vi "TemperatureConverter.vi"() -> ()   [LabVIEW 2021]
panel:
  in  "(STOP)":bool
  out "Output":dbl
  in  "Input":dbl
  in  "MODE":T1(ring)
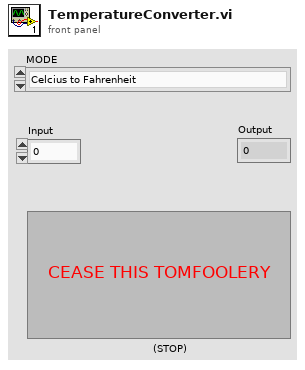
[diagram p1: front panel]
types:
  T1 = enum16{"Celcius to Fahrenheit", "Fahrenheit to Celcius", "Celcius to Kelvin", "Fahrenheit to Kelvin"}
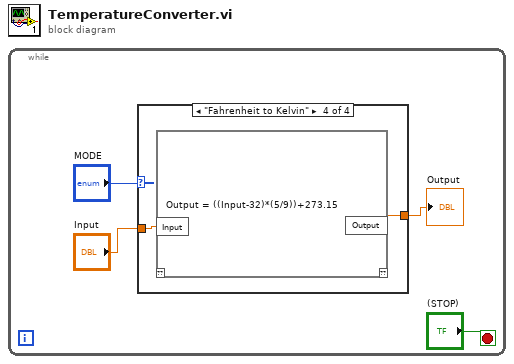
[diagram p0: block diagram]
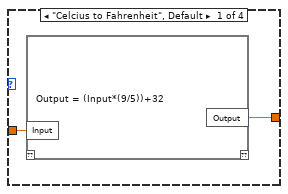
[diagram p2: hidden frame]
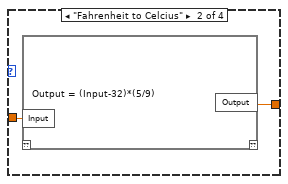
[diagram p3: hidden frame]
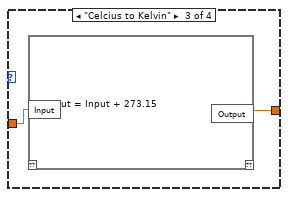
[diagram p4: hidden frame]
diagram:
  n1 = while {
    stop <- "(STOP)" stop-if-true
    n2 = case shown="\"Fahrenheit to Kelvin\"" "MODE" {
      tunnel: [w6 w8 w10 w12] -> w2
      tunnel: "Input" -> [w5 w7 w9 w11]
      frame "Celcius to Fahrenheit", Default {
        n3 = script code="Output = (Input*(9/5))+32"("Input"=w5) -> ("Output"=w6:dbl)  [unwired: 1 in, 1 out]
      }
      frame "Fahrenheit to Celcius" {
        n4 = script code="Output = (Input-32)*(5/9)"("Input"=w7) -> ("Output"=w8:dbl)  [unwired: 1 in, 1 out]
      }
      frame "Celcius to Kelvin" {
        n5 = script code="Output = Input + 273.15"("Input"=w9) -> ("Output"=w10:dbl)  [unwired: 1 in, 1 out]
      }
      frame "Fahrenheit to Kelvin" {
        n6 = script code="Output = ((Input-32)*(5/9))+273.15"("Input"=w11) -> ("Output"=w12:dbl)  [unwired: 1 in, 1 out]
      }
    }
    "Output" <- w2
  }
